vi "ImagePretreat.vi"(0 "Image Src":T2, 1 "error in (no error)":errorcluster) -> (2 "灰度直方图":T1(graph), 3 "Image Dst Out":T2, 4 "error out":errorcluster)   [LabVIEW 2012]
uses:
  <vilib>/vision/Image Controls.llb/IMAQ Image.ctl
  <vilib>/vision/NI_Vision_Development_Module.lvlib
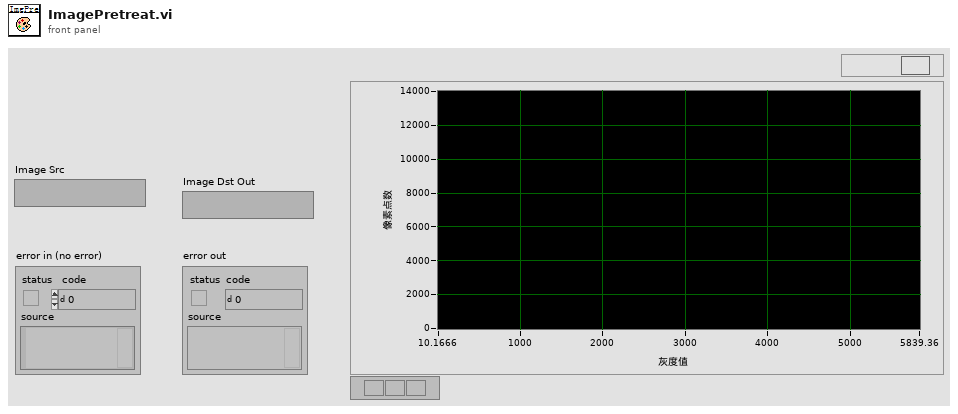
[diagram p1: front panel]
types:
  T1 = cluster{"Starting Value":sgl, "Incremental Value":sgl, "Histogram":u32[]}
  T2 = typedef "IMAQ Image.ctl" = refnum<image>
  T3 = enum32{"AutoM", "Close", "Dilate", "Erode", "Gradient", "Gradient in", "Gradient out", "HitMiss", "Open", "PClose", "POpen", "Thick", "Thin"}
  T4 = typedef "Image Type" = u32
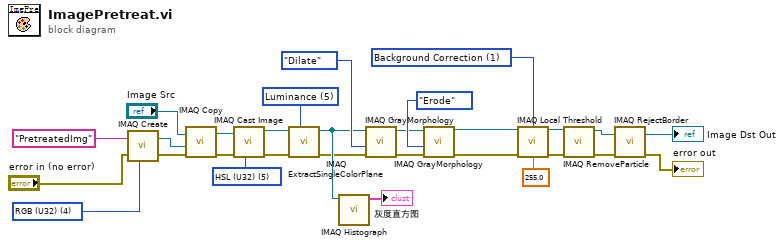
[diagram p0: block diagram]
diagram:
  w15 = u32 1 items=["Niblack", "Background Correction"] ("Method (Niblack)")
  w18 = T4 4 items=["Grayscale (U8)", "Grayscale (I16)", "Grayscale (SGL)", "Complex (CSG)", "RGB (U32)", "HSL (U32)", "RGB (U64)", "Grayscale (U16)"] ("Image Type")
  w19 = 5 items=["Red", "Green", "Blue", "Hue", "Saturation", "Luminance", "Value", "Intensity"] ("Color Plane")
  w24 = T4 5 items=["Grayscale (U8)", "Grayscale (I16)", "Grayscale (SGL)", "Complex (CSG)", "RGB (U32)", "HSL (U32)", "RGB (U64)", "Grayscale (U16)"] ("Image Type")
  n1 = call "IMAQ Create"("Image Name"="PretreatedImg", "Image Type"=w18, "error in (no error)"="error in (no error)") -> ("New Image"=w26:T2, "error out"=w27:errorcluster)  [unwired: 2 in]
  n2 = call "IMAQ Copy"("error in (no error)"=w27, "Image Dst"=w26, "Image Src"="Image Src") -> ("error out"=w20:errorcluster, "Image Dst Out"=w21:T2)  [unwired: 3 in]
  n3 = call "IMAQ Cast Image"("Image Type"=w24, "error in (no error)"=w20, "Image Src"=w21) -> ("error out"=w22:errorcluster, "Image Dst Out"=w23:T2)  [unwired: 7 in]
  n4 = call "IMAQ ExtractSingleColorPlane"("Color Plane"=w19, "error in (no error)"=w22, "Image Src"=w23) -> ("error out"=w12:errorcluster, "Image Dst Out"=w13:T2)  [unwired: 7 in]
  n5 = call "IMAQ Histograph"("Image"=w13) -> ("Histogram Graph"=→"灰度直方图":T1)  [unwired: 7 in, 3 out]
  n6 = call "IMAQ GrayMorphology"("error in (no error)"=w12, "Operation"=T3."Dilate", "Image Src"=w13) -> ("error out"=w9:errorcluster, "Image Dst Out"=w10:T2)  [unwired: 7 in]
  n7 = call "IMAQ GrayMorphology"("error in (no error)"=w9, "Operation"=T3."Erode", "Image Src"=w10) -> ("error out"=w8:errorcluster, "Image Dst Out"=w7:T2)  [unwired: 7 in]
  n8 = call "IMAQ Local Threshold"("Image Src"=w7, "Method (Niblack)"=w15, "error in (no error)"=w8, "Replace Value (1)"=sgl 255.0) -> ("Image Dst Out"=w6:T2, "error out"=w5:errorcluster)  [unwired: 10 in]
  n9 = call "IMAQ RemoveParticle"("error in (no error)"=w5, "Image Src"=w6) -> ("error out"=w3:errorcluster, "Image Dst Out"=w4:T2)  [unwired: 8 in]
  n10 = call "IMAQ RejectBorder"("error in (no error)"=w3, "Image Src"=w4) -> ("error out"=→"error out":errorcluster, "Image Dst Out"=→"Image Dst Out":T2)  [unwired: 4 in]
